vi "Telescope Configure GUI.vi"(8 "error in (no error)":errorcluster, 10 "Telescope Name":string="PRIME", 11 "PRIME Telescope in":refnum<class "PRIME Telescope.lvclass">) -> (0 "error out":errorcluster, 3 "PRIME Telescope out":refnum<class "PRIME Telescope.lvclass">)   [LabVIEW 2021, in "PRIME Telescope.lvclass"]
uses:
  PRIME Telescope.lvclass
  PRIME Telescope.lvclass/PRIME Telescope.ctl
  Telescope.lvclass
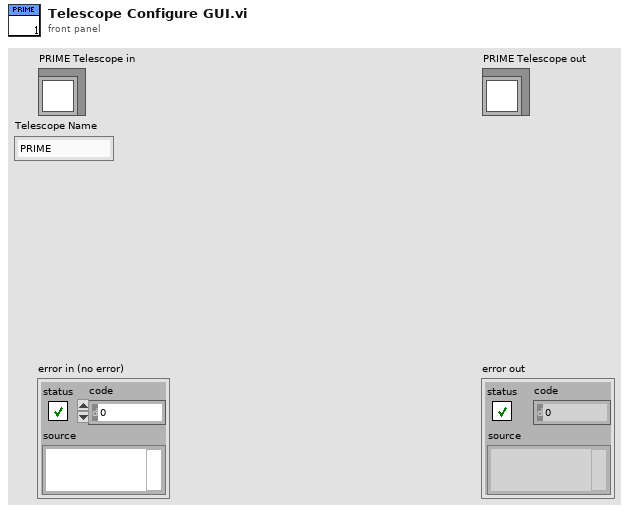
[diagram p1: front panel]
types:
  T1 = typedef "PRIME Telescope cluster Settings.ctl" = cluster{"IP Address":string, "port":u16}
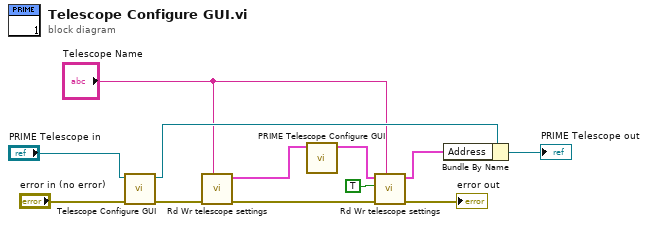
[diagram p0: block diagram]
diagram:
  n1 = call-parent "Telescope Configure GUI.vi"("error in (no error)"="error in (no error)", "Telescope in"="PRIME Telescope in") -> ("error out"=w9:errorcluster, "Telescope out"=w8:refnum<class "PRIME Telescope.lvclass">)  [unwired: 8 in]
  n2 = call "Rd Wr telescope settings.vi"("Telescope Name"="Telescope Name", "error in (no error)"=w9) -> ("error out"=w5:errorcluster, "Telescope Settings"=w7:T1)  [unwired: 8 in]
  n3 = call "PRIME Telescope Configure GUI.vi"("Settings"=w7) -> ("Settings out"=w2:T1)  [unwired: 10 in]
  n4 = call "Rd Wr telescope settings.vi"("Telescope Name"="Telescope Name", "error in (no error)"=w5, "Write? (F:Read)"=TRUE, "Telescope Settings"=w2) -> ("error out"=→"error out":errorcluster, "Telescope Settings"=w3:T1)  [unwired: 6 in]
  n5 = Bundle By Name(cluster=w8, "Address"=w3) -> (→"PRIME Telescope out":refnum<class "PRIME Telescope.lvclass">)
